vi "voltageSet_backup.vi"(3 "error in (no error)":errorcluster, 4 "Voltage":dbl=0.5 min=0.5 max=20.0, 5 "I2c Port in":u8=1) -> (0 "error out":errorcluster, 1 "Numeric":dbl, 2 "I2c Port out":u8)   [LabVIEW 2016]
uses:
  VIs/ControlI2C.lvlib
panel:
  out "unsigned byte array":u8[](array[numeric])
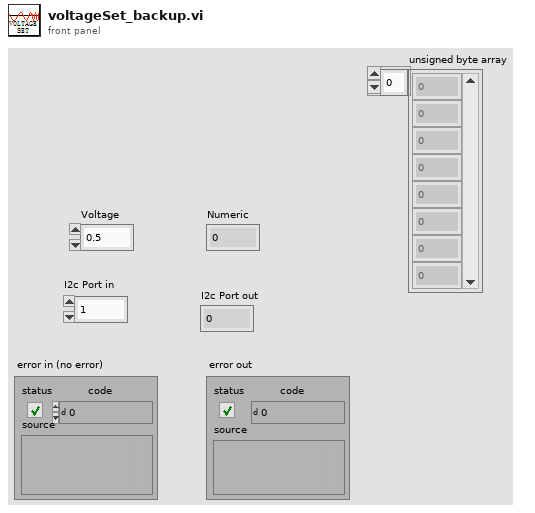
[diagram p1: front panel]
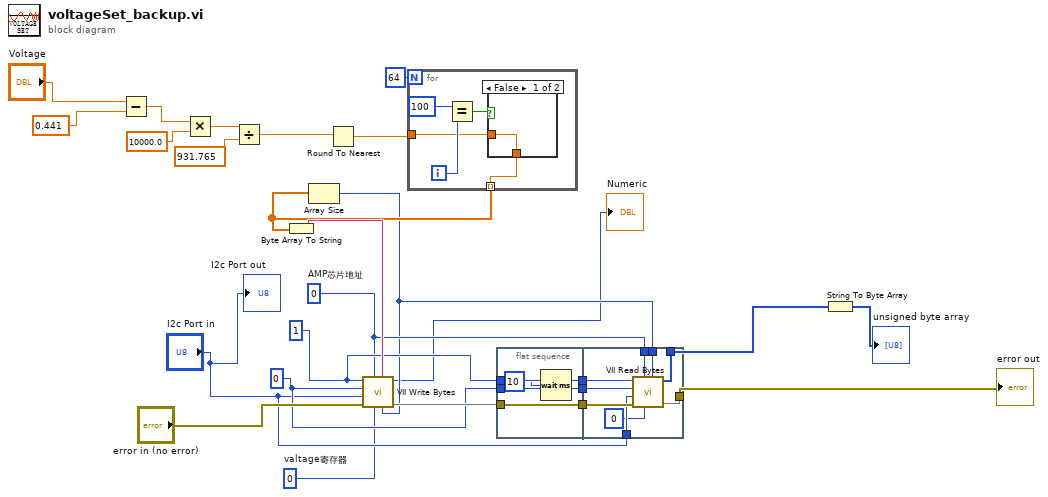
[diagram p0: block diagram]
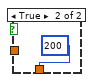
[diagram p2: hidden frame]
diagram:
  w7 = u8 0  # valtage寄存器
  w6 = u8 0  # AMP芯片地址
  w9 = 0
  w10 = 1
  n1 = Subtract(x="Voltage", y=0.441) -> (x-y=w21:dbl)
  n2 = Multiply(x=w21, y=10000.0) -> (x*y=w19:dbl)
  n3 = Divide(x=w19, y=931.765) -> (x/y=w16:dbl)
  n4 = Round To Nearest(number=w16) -> (nearest integer value=w15:dbl)
  n5 = for {
    N: 64 -> [_]
    tunnel: w15 -> [w28]
    tunnel: [w27] -> w17 mode=indexing
    i -> [w31]
    n6 = Equal?(x=100, y=w31) -> (x = y?=w29:bool)
    n7 = case shown="False" w29 {
      tunnel: w28 -> [w32 _]
      tunnel: [w32 200] -> w27
      frame False {
      }
      frame True {
      }
    }
  }
  n8 = Byte Array To String(unsigned byte array=w17) -> (string=w25:string)
  n9 = Array Size(array=w17) -> (size(s)=w5:i32)
  n10 = call "VII Write Bytes.vi"("Len"=w5, 5:w25, "SubAddr"=w7, "SlaveAddr"=w6, 8:"error in (no error)", "I2CIndex"="I2c Port in", "DevIndex"=w9, "DevType"=w10) -> (0:w14, "function return"=→"Numeric":i32)  [unwired: 2 in]
  n11 = flat-sequence {
    tunnel: w9 -> [w35]
    tunnel: w10 -> [w36]
    tunnel: w14 -> [w37]
    tunnel: [w37] -> w4
    tunnel: [w36] -> w3
    tunnel: [w35] -> w2
    tunnel: [w45] -> w13
    tunnel: [w44] -> w12
    tunnel: "I2c Port in" -> [w41]
    tunnel: w6 -> [w40]
    tunnel: w5 -> [w39]
    tunnel: w4 -> [w46]
    tunnel: w3 -> [w43]
    tunnel: w2 -> [w42]
    frame #0 {
      n12 = Wait (ms)(milliseconds to wait=u32 10) -> ()  [unwired: 1 out]
    }
    frame #1 {
      n13 = call "VII Read Bytes.vi"("Len"=w39, "SubAddr"=0, "SlaveAddr"=w40, 8:w46, "I2CIndex"=w41, "DevIndex"=w42, "DevType"=w43) -> (0:w45, "pReadData"=w44:u8[])  [unwired: 2 in, 1 out]
    }
  }
  n14 = String To Byte Array(string=w12) -> (unsigned byte array=→"unsigned byte array":u8[])
  "I2c Port out" <- "I2c Port in"
  "error out" <- w13
